vi "Addressed to This Module.vi"(10 "Module ID from Argument":i32, 11 "Module Admin":refnum<class "Delacor_lib_QMH_Cloneable Module Admin.lvclass">) -> (1 "Addressed to ALL (-1) ?":bool, 3 "Addressed to this instance?":bool)   [LabVIEW 2019, in "moduloDqmh.lvlib"]
doc: "Determine if the module ID returned in an event argument is intended for this specific cloneable module instance.\n_____\nBased on Delacor QMH Project Template 5.0.0.82."
uses:
  moduloDqmh.lvlib
  <vilib>/Delacor/Delacor QMH/Libraries/Cloneable Module Admin_class/Delacor_lib_QMH_Cloneable Module Admin.lvclass
  <vilib>/Delacor/Delacor QMH/Libraries/Cloneable Module Admin_class/Delacor_lib_QMH_Cloneable Module Admin.lvclass/Delacor_lib_QMH_Cloneable Module Admin.ctl
  <vilib>/Delacor/Delacor QMH/Libraries/Cloneable Module Admin_class/Delacor_lib_QMH_Get Module ID.vi
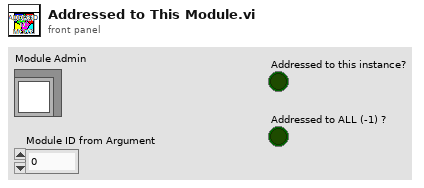
[diagram p1: front panel]
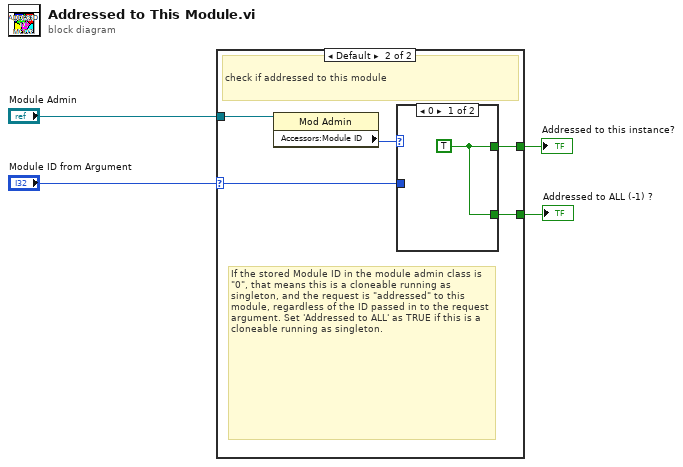
[diagram p0: block diagram]
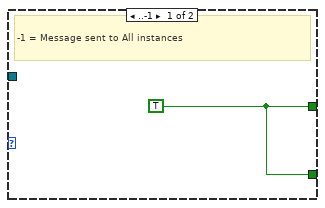
[diagram p2: hidden frame]
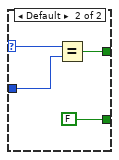
[diagram p3: hidden frame]
diagram:
  n1 = case shown="Default" "Module ID from Argument" {
    selector: "Module ID from Argument" -> [_ w9]
    tunnel: [w5 w10] -> w4
    tunnel: "Module Admin" -> [_ w8]
    tunnel: [w5 w6] -> w1
    frame ..-1 {
      w5 = TRUE
      # "-1 = Message sent to All instances"
    }
    frame Default {
      # "If the stored Module ID in the module admin class is \"0\", that means this is a cloneable running as singleton, and the request is \"addressed\" to this module, regardless of the ID passed in to the request argument. Set 'Addressed to ALL' as TRUE if this is a cloneable running as singleton."
      # "check if addressed to this module"
      n2 = property class="Mod Admin"(reference=w8) -> ("Accessors:Module ID"=w7:i32)  [unwired: 1 in, 2 out]
      n3 = case shown="0" w7 {
        selector: w7 -> [_ w13]
        tunnel: [w11 w15] -> w10
        tunnel: w9 -> [_ w14]
        tunnel: [w11 FALSE] -> w6
        frame 0 {
          w11 = TRUE
        }
        frame Default {
          n4 = Equal?(x=w13, y=w14) -> (x = y?=w15:bool)
        }
      }
    }
  }
  "Addressed to this instance?" <- w4
  "Addressed to ALL (-1) ?" <- w1
